vi "Register_Unregister_UserEvents_PSMGUI.vi"(0 "Event Registration Refnum IN":refnum<event-registration>, 1 "Action":enum16{"Register", "Un-Register"}(ring), 5 "Pos X IN":dbl, 7 "Pos Y IN":dbl, 9 "Pos Z IN":dbl, 11 "error in (no error)":errorcluster) -> (4 "Event Registration Refnum OUT":refnum<event-registration>, 6 "Pos X OUT":dbl, 8 "Pos Y OUT":dbl, 10 "Pos Z  OUT":dbl, 15 "error out":errorcluster)   [LabVIEW 2012]
doc: "SciScan 1.2 160622"
uses:
  <vilib>/Utility/VariantDataType/Type.ctl
  Image Validity FGV_Commands.ctl
  <vilib>/Utility/VariantDataType/VariantType.lvlib
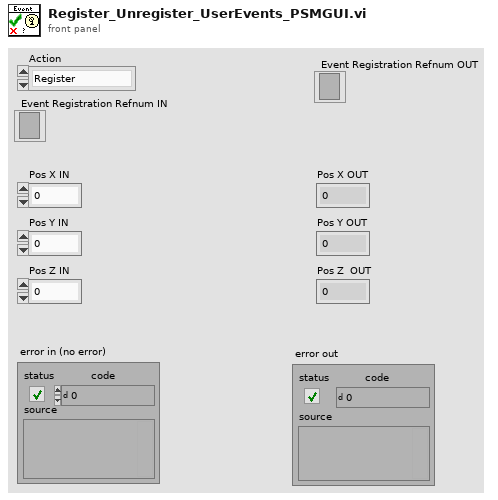
[diagram p1: front panel]
types:
  T1 = typedef "Image Validity FGV_Commands.ctl" = enum16{"Set validity status", "Get Validity status"}
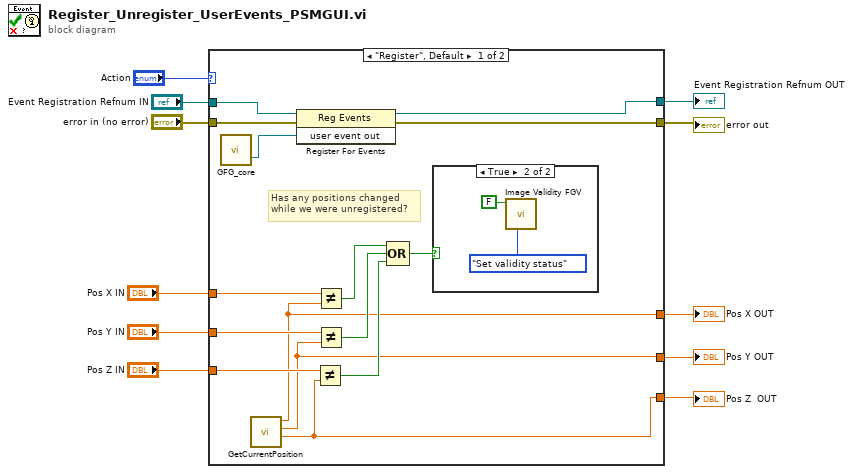
[diagram p0: block diagram]
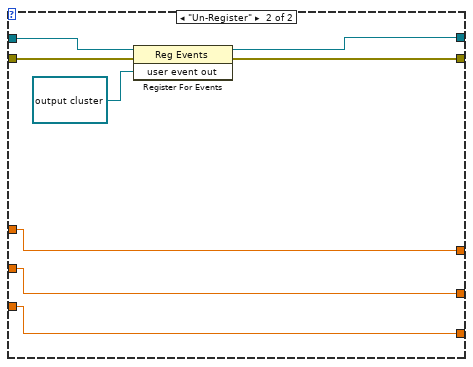
[diagram p3: hidden frame]
diagram:
  n1 = case shown="\"Register\", Default" "Action" {
    tunnel: "Event Registration Refnum IN" -> [w26 w36]
    tunnel: [w23 w34] -> w8
    tunnel: [w22 w33] -> w7
    tunnel: "error in (no error)" -> [w24 w32]
    tunnel: "Pos X IN" -> [w21 w31]
    tunnel: "Pos Y IN" -> [w20 w30]
    tunnel: "Pos Z IN" -> [w19 w29]
    tunnel: [w15 w31] -> w3
    tunnel: [w14 w30] -> w2
    tunnel: [w13 w29] -> w1
    frame "Register", Default {
      # "Has any positions changed\nwhile we were unregistered?"
      n2 = call "GFG_core.vi"() -> ("user event out"=w25:refnum<user-event>)  [unwired: 13 in, 6 out]
      n3 = call "GetCurrentPosition.vi"() -> ("Z"=w13:dbl, "Y"=w14:dbl, "X"=w15:dbl)  [unwired: 8 in, 1 out]
      n4 = register-events(reference=w26, error in=w24, w25) -> (reference out=w22:refnum<event-registration>, error out=w23:errorcluster)
      n5 = Not Equal?(x=w19, y=w13) -> (x != y?=w16:bool)
      n6 = Not Equal?(x=w21, y=w15) -> (x != y?=w18:bool)
      n7 = Not Equal?(x=w20, y=w14) -> (x != y?=w17:bool)
      n8 = Compound Arithmetic op=OR(w18, w17, w16) -> (w12:bool)
      n9 = case shown="True" w12 {
        frame False {
        }
        frame True {
          n10 = call "Image Validity FGV.vi"("Image Validity FGV_Commands"=Image_Validity_FGV_Commands."Set validity status", "Validity status IN"=FALSE) -> ()  [unwired: 8 in, 2 out]
        }
      }
    }
    frame "Un-Register" {
      n11 = register-events(reference=w36, error in=w32, refnum<user-event> refnum ("event source")) -> (reference out=w33:refnum<event-registration>, error out=w34:errorcluster)
    }
  }
  "error out" <- w8
  "Event Registration Refnum OUT" <- w7
  "Pos Y OUT" <- w2
  "Pos Z  OUT" <- w1
  "Pos X OUT" <- w3
